vi "AdvFilter-Init.vi"(5 "Filter":T1 {"Stages"."IIR Filter"."Forward Coefficients" format="%.4f"; "Stages"."IIR Filter"."Reverse Coefficients" format="%.4f"}, 9 "Sampling rate (Hz)":dbl, 11 "error in (no error)":errorcluster) -> (6 "Filter out":T1 {"Stages"."IIR Filter"."Forward Coefficients" format="%.4f"; "Stages"."IIR Filter"."Reverse Coefficients" format="%.4f"}, 15 "error out":errorcluster)   [LabVIEW 2020]
uses:
  Controls/Advanced Filter XCtl/Filter Data.ctl
  Filter-Bandwidth Units.ctl
  <vilib>/Analysis/3filter.llb/Filter Passband Type.ctl
  <vilib>/Analysis/NI_AALBase.lvlib
  Controls/Advanced Filter XCtl/Advanced Filter XCtl.xctl
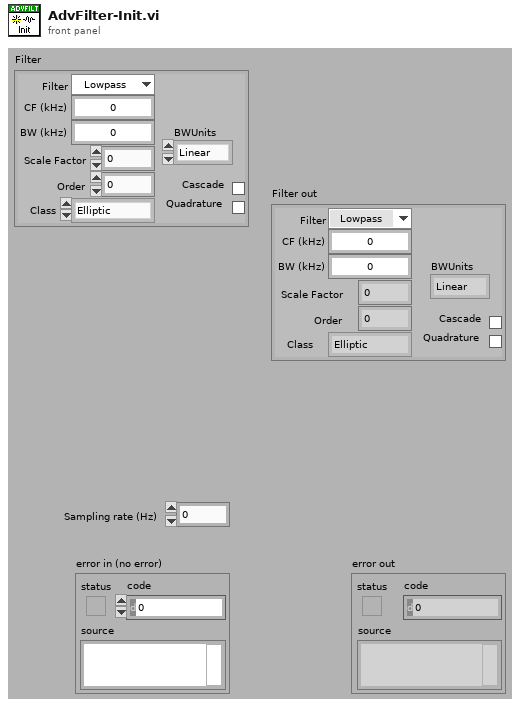
[diagram p1: front panel]
types:
  T1 = typedef "Advanced Filter XCtl.xctl/Filter Data.ctl" = cluster{"Type":enum16{"Lowpass", "Highpass", "Bandpass", "Bandstop", "OFF"}, "CF (kHz)":dbl, "BW (kHz)":dbl, "Cascade":bool, "Quadrature":bool, "Scale Factor":dbl, "Stages":cluster{"IIR Filter":cluster{"filter structure":enum32{"IIR 2nd Order", "IIR 4th Order"}, "Reverse Coefficients":dbl[], "Forward Coefficients":dbl[]}, "State":dbl[]}[], "Class":enum16{"Elliptic", "Butterworth"}, "Order":i32, "BWUnits":T2}
  T2 = typedef "Filter-Bandwidth Units.ctl" = enum16{"Linear", "Octaves", "Min-Max"}
  T3 = enum16{"Lowpass", "Highpass", "Bandpass", "Bandstop", "OFF"}
  T4 = cluster{"IIR Filter Cluster":cluster{"filter structure":enum32{"IIR 2nd Order", "IIR 4th Order"}, "Reverse Coefficients":dbl[], "Forward Coefficients":dbl[]}, "Final Filter State":dbl[]}[]
  T5 = typedef "NI_AALBase.lvlib/Filter Passband Type.ctl" = enum32{"Lowpass", "Highpass", "Bandpass", "Bandstop"}
  T6 = cluster{"IIR Filter Cluster":cluster{"filter structure":enum32{"IIR 2nd Order", "IIR 4th Order"}, "Reverse Coefficients":dbl[], "Forward Coefficients":dbl[]}, "Final Filter State":dbl[]}
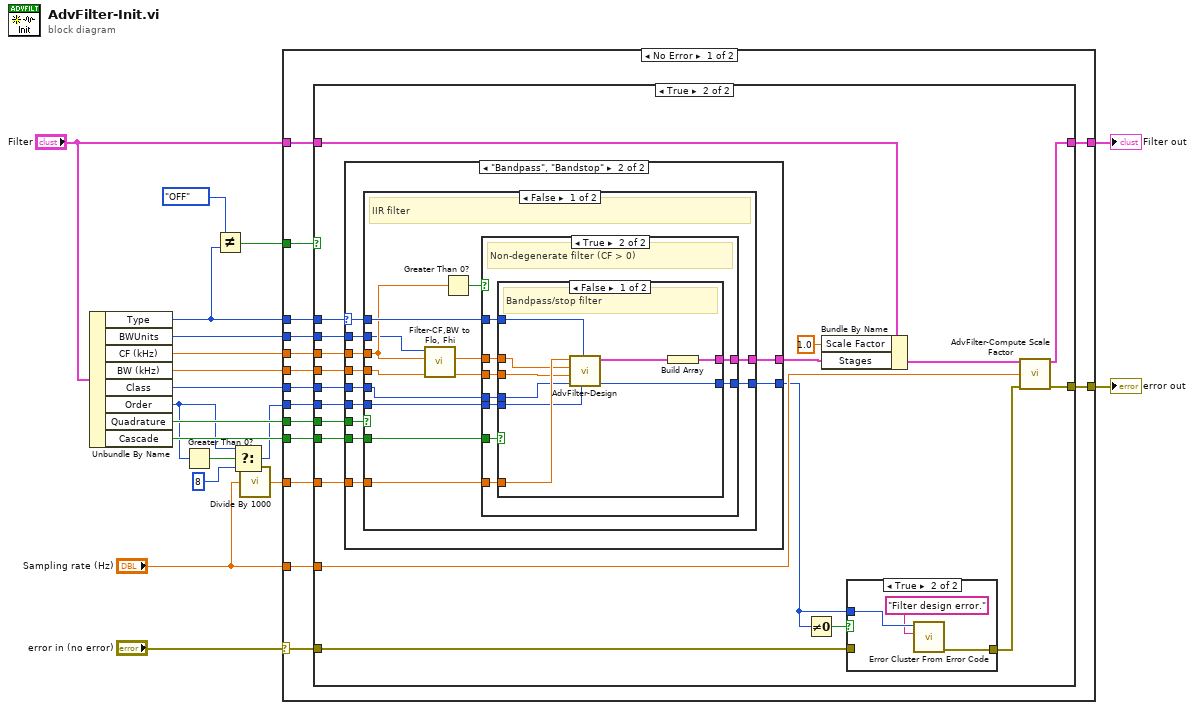
[diagram p0: block diagram]
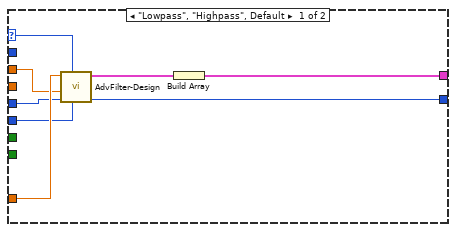
[diagram p4: hidden frame]
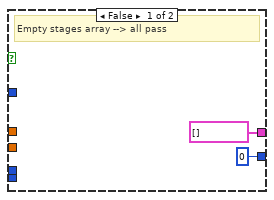
[diagram p5: hidden frame]
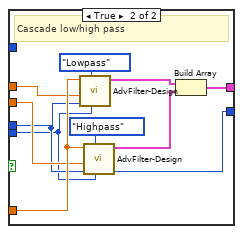
[diagram p6: hidden frame]
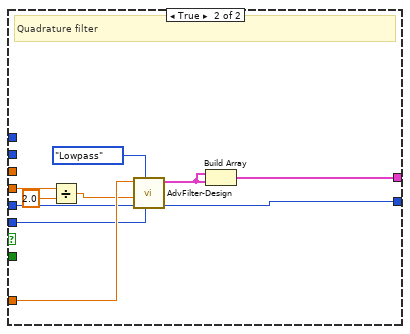
[diagram p7: hidden frame]
diagram:
  n1 = Unbundle By Name("Filter") -> ("Type"=w6:T3, "BWUnits"=w5:T2, "CF (kHz)"=w16:dbl, "BW (kHz)"=w15:dbl, "Class"=w10:enum16{"Elliptic", "Butterworth"}, "Order"=w2:i32, "Quadrature"=w13:bool, "Cascade"=w9:bool)
  n2 = Greater Than 0?(x=w2) -> (x > 0?=w4:bool)
  n3 = Not Equal?(x=T3."OFF", y=w6) -> (x != y?=w11:bool)
  n4 = Select(t=w2, s=w4, f=8) -> (s? t:f=w3:i32)
  n5 = call "Divide By 1000.vi"("X"="Sampling rate (Hz)") -> ("X/1000"=w7:dbl)
  n6 = case shown="No Error" "error in (no error)" {
    selector: "error in (no error)" -> [w27 w134]
    tunnel: w11 -> [w34 _]
    tunnel: w6 -> [w33 _]
    tunnel: "Sampling rate (Hz)" -> [w32 _]
    tunnel: "Filter" -> [w31 w135]
    tunnel: [w30 w135] -> w17
    tunnel: w16 -> [w29 _]
    tunnel: w15 -> [w28 _]
    tunnel: [w26 w134] -> w14
    tunnel: w13 -> [w25 _]
    tunnel: w10 -> [w24 _]
    tunnel: w3 -> [w23 _]
    tunnel: w7 -> [w22 _]
    tunnel: w9 -> [w21 _]
    tunnel: w5 -> [w20 _]
    frame No Error {
      n7 = case shown="True" w34 {
        tunnel: w33 -> [_ w50]
        tunnel: w32 -> [_ w51]
        tunnel: w31 -> [w36 w56]
        tunnel: [w36 w41] -> w30
        tunnel: w29 -> [_ w55]
        tunnel: w28 -> [_ w54]
        tunnel: w27 -> [w35 w52]
        tunnel: [w35 w38] -> w26
        tunnel: w25 -> [_ w49]
        tunnel: w24 -> [_ w48]
        tunnel: w23 -> [_ w47]
        tunnel: w22 -> [_ w45]
        tunnel: w21 -> [_ w43]
        tunnel: w20 -> [_ w37]
        frame False {
        }
        frame True {
          n8 = case shown="\"Bandpass\", \"Bandstop\"" w50 {
            selector: w50 -> [w67 w70]
            tunnel: w55 -> [w61 w78]
            tunnel: w54 -> [_ w79]
            tunnel: w49 -> [_ w77]
            tunnel: w48 -> [w66 w74]
            tunnel: w47 -> [w65 w75]
            tunnel: [w63 w72] -> w46
            tunnel: w45 -> [w68 w76]
            tunnel: [w62 w73] -> w44
            tunnel: w43 -> [_ w71]
            tunnel: w37 -> [_ w69]
            frame "Lowpass", "Highpass", Default {
              n9 = call "AdvFilter-Design.vi"("order"=w65, "filter type"=w67, "Class"=w66, "low cutoff freq: fl"=w61, "sampling freq: fs"=w68) -> ("error"=w62:i32, "IIR Filter"=w64:T6)  [unwired: 5 in]
              n10 = Build Array(w64) -> (w63:T4)
            }
            frame "Bandpass", "Bandstop" {
              n11 = case shown="False" w77 {
                tunnel: w79 -> [w82 w133]
                tunnel: w78 -> [w85 _]
                tunnel: w76 -> [w90 w130]
                tunnel: w75 -> [w89 w129]
                tunnel: w74 -> [w88 w128]
                tunnel: [w86 w126] -> w73
                tunnel: [w87 w124] -> w72
                tunnel: w71 -> [w92 _]
                tunnel: w70 -> [w91 _]
                tunnel: w69 -> [w83 _]
                frame False {
                  # "IIR filter"
                  n12 = call "Filter-CF,BW to Flo, Fhi.vi"("BW"=w82, "CF (kHz)"=w85, "BWUnits"=w83) -> ("Fmin"=w80:dbl, "Fmax"=w81:dbl)  [unwired: 7 in]
                  n13 = Greater Than 0?(x=w85) -> (x > 0?=w84:bool)
                  n14 = case shown="True" w84 {
                    tunnel: w92 -> [_ w103]
                    tunnel: w91 -> [_ w102]
                    tunnel: w90 -> [_ w101]
                    tunnel: w81 -> [_ w100]
                    tunnel: w80 -> [_ w99]
                    tunnel: w89 -> [_ w98]
                    tunnel: w88 -> [_ w97]
                    tunnel: [T4 [] w96] -> w87
                    tunnel: [0 ("error") w95] -> w86
                    frame False {
                      # "Empty stages array --> all pass"
                    }
                    frame True {
                      # "Non-degenerate filter (CF > 0)"
                      n15 = case shown="False" w103 {
                        tunnel: w102 -> [w112 _]
                        tunnel: w101 -> [w111 w123]
                        tunnel: w100 -> [w110 w122]
                        tunnel: w99 -> [w109 w121]
                        tunnel: w98 -> [w108 w113]
                        tunnel: w97 -> [w107 w114]
                        tunnel: [w106 w117] -> w96
                        tunnel: [w104 w115] -> w95
                        frame False {
                          # "Bandpass/stop filter"
                          n16 = call "AdvFilter-Design.vi"("order"=w108, "filter type"=w112, "Class"=w107, "low cutoff freq: fl"=w109, "high cutoff freq: fh"=w110, "sampling freq: fs"=w111) -> ("error"=w104:i32, "IIR Filter"=w105:T6)  [unwired: 4 in]
                          n17 = Build Array(w105) -> (w106:T4)
                        }
                        frame True {
                          # "Cascade low/high pass"
                          n18 = call "AdvFilter-Design.vi"("order"=w113, "filter type"=Filter_Passband_Type."Lowpass", "Class"=w114, "low cutoff freq: fl"=w122, "sampling freq: fs"=w123) -> ("IIR Filter"=w118:T6)  [unwired: 5 in, 1 out]
                          n19 = call "AdvFilter-Design.vi"("order"=w113, "filter type"=Filter_Passband_Type."Highpass", "Class"=w114, "low cutoff freq: fl"=w121, "sampling freq: fs"=w123) -> ("error"=w115:i32, "IIR Filter"=w116:T6)  [unwired: 5 in]
                          n20 = Build Array(w118, w116) -> (w117:T4)
                        }
                      }
                    }
                  }
                }
                frame True {
                  # "Quadrature filter"
                  n21 = Divide(x=w133, y=2.0) -> (x/y=w127:dbl)
                  n22 = call "AdvFilter-Design.vi"("order"=w129, "filter type"=Filter_Passband_Type."Lowpass", "Class"=w128, "low cutoff freq: fl"=w127, "sampling freq: fs"=w130) -> ("error"=w126:i32, "IIR Filter"=w125:T6)  [unwired: 5 in]
                  n23 = Build Array(w125, w125) -> (w124:T4)
                }
              }
            }
          }
          n24 = Not Equal To 0?(x=w44) -> (x != 0?=w53:bool)
          n25 = Bundle By Name(cluster=w56, "Scale Factor"=1.0, "Stages"=w46) -> (w42:T1)
          n26 = case shown="True" w53 {
            tunnel: [w57 w59] -> w39
            tunnel: w52 -> [w57 _]
            tunnel: w44 -> [_ w60]
            frame False {
            }
            frame True {
              n27 = call <vilib>:"Error Cluster From Error Code.vi"("error message (\"\")"="Filter design error." ("error message (\"\")"), "error code (0)"=w60) -> ("error out"=w59:errorcluster)  [unwired: 7 in]
            }
          }
          n28 = call "AdvFilter-Compute Scale Factor.vi"("Filter"=w42, "Sampling Rate (Hz)"=w51, "error in (no error)"=w39) -> ("Filter out"=w41:T1, "error out"=w38:errorcluster)  [unwired: 11 in]
        }
      }
    }
    frame Error {
    }
  }
  "error out" <- w14
  "Filter out" <- w17
